vi "Read Keys.vi"(8 "error in (no error)":errorcluster, 11 "Section 2a in":refnum<class "Section 2a.lvclass">) -> (0 "error out":errorcluster, 2 "Keys":cluster{"Name":string, "Value":string}[](array[cluster]), 3 "Section 2a out":refnum<class "Section 2a.lvclass">)   [LabVIEW 2012, in "LVOOP Introduction.lvlib" / "Section 2a.lvclass"]
doc: "Thi VI returns an array of key/values pairs of section.\n\nOverwriting dynamic dispatch VI."
uses:
  Section 2a.lvclass
  Section 2/Section 2.lvclass
  Read I32.vi
  Read U32.vi
  Read Path.vi
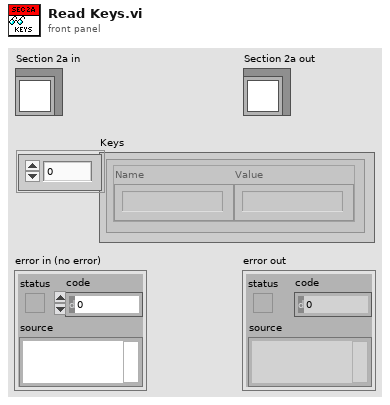
[diagram p1: front panel]
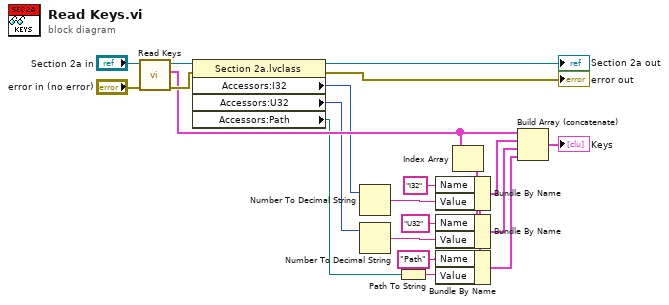
[diagram p0: block diagram]
diagram:
  n1 = call-parent "Read Keys.vi"("error in (no error)"="error in (no error)", "Section 2 in"="Section 2a in") -> ("error out"=w9:errorcluster, "Keys"=w8:cluster{"Name":string, "Value":string}[], "Section 2 out"=w12:refnum<class "Section 2a.lvclass">)  [unwired: 7 in]
  n2 = property class="Section 2a.lvclass"(reference=w12, error in=w9) -> (reference out=→"Section 2a out":refnum<class "Section 2a.lvclass">, error out=→"error out":errorcluster, "Accessors:I32"=w5:i32, "Accessors:U32"=w2:u32, "Accessors:Path"=w6:path)
  n3 = Number To Decimal String(number=w5) -> (decimal integer string=w4:string)  [unwired: 1 in]
  n4 = Number To Decimal String(number=w2) -> (decimal integer string=w3:string)  [unwired: 1 in]
  n5 = Path To String(path=w6) -> (string=w7:string)
  n6 = Index Array(array=w8) -> (element=w19:cluster{"Name":string, "Value":string})  [unwired: 1 in]
  n7 = Bundle By Name(cluster=w19, "Name"="Path", "Value"=w7) -> (w13:cluster{"Name":string, "Value":string})
  n8 = Bundle By Name(cluster=w13, "Name"="U32", "Value"=w3) -> (w14:cluster{"Name":string, "Value":string})
  n9 = Bundle By Name(cluster=w14, "Name"="I32", "Value"=w4) -> (w15:cluster{"Name":string, "Value":string})
  n10 = Build Array (concatenate)(w8, w15, w14, w13) -> (→"Keys":cluster{"Name":string, "Value":string}[])
